vi "Main Page.vi"(8 "error in (no error)":errorcluster, 11 "Node Ptr":T1 format="%.0x") -> (0 "error out":errorcluster)   [LabVIEW 2020, in "NI PXIe-4340 System Explorer.lvlib"]
uses:
  NI PXIe-4340 System Explorer.lvlib
  <vilib>/NI VeriStand/Custom Device API/Custom Device Item Ref.ctl
  Shared/Constants.vi
  <vilib>/NI VeriStand/Custom Device API/Set Item Property (String).vi
  <vilib>/NI VeriStand/Custom Device API/Set Item Property (Double).vi
  <vilib>/NI VeriStand/Custom Device API/Set Item Property (Variant).vi
  <vilib>/NI VeriStand/Custom Device API/Custom Device API.lvlib
  Shared/NI PXIe-4340 Shared.lvlib
panel:
  in  "Sample Rate (Hz)":dbl
  in  "Device Name":string
  in  "Configure Physical Channels":bool
  in  "Header":cluster{"Section Name":string}={"Section Name"="Custom Device Item Settings"}
  in  "Description":string
  in  "Name":string
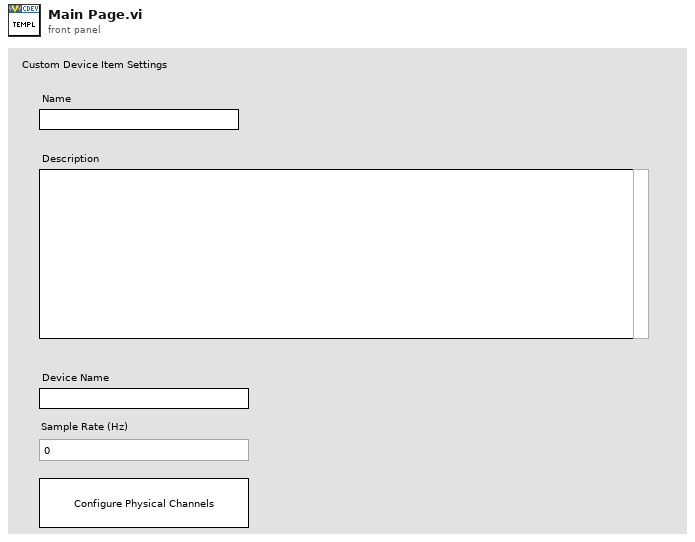
[diagram p1: front panel]
types:
  T1 = typedef "Custom Device API.lvlib/Custom Device Item Ref.ctl" = u64
  T2 = typedef "Custom Device API.lvlib/Custom Device Item Info.ctl" = cluster{"Name":string, "Is Channel":bool, "GUID":string, "Is Waveform":bool}
  T3 = typedef "NI PXIe-4340 Shared.lvlib/Device Configuration.ctl" = cluster{"Task":refnum<k21>, "Device Name":string, "Sample Rate (Hz)":dbl, "Enabled Channels":bool[]}
  T4 = typedef "Custom Device API.lvlib/Custom Device Commands.ctl" = enum16{"Default", "Item renamed", "Shutdown", "Dynamic button pressed"}
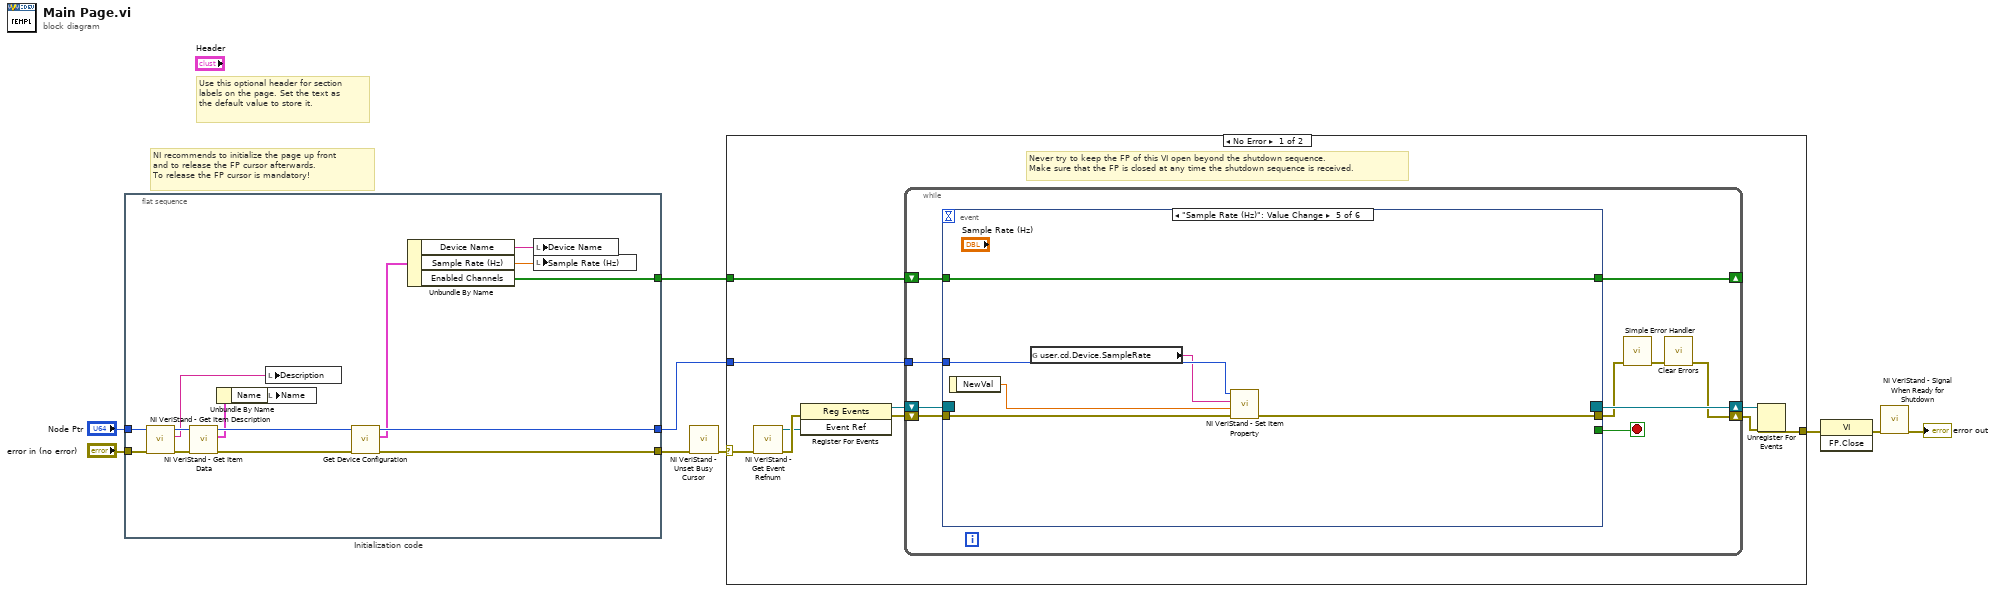
[diagram p0: block diagram]
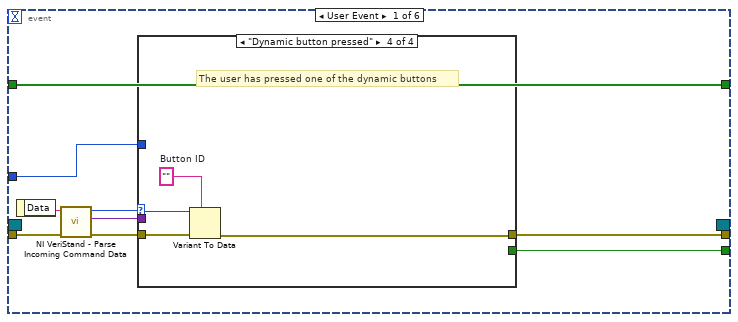
[diagram p2: hidden frame]
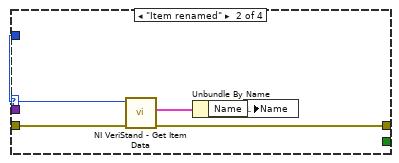
[diagram p4: hidden frame]
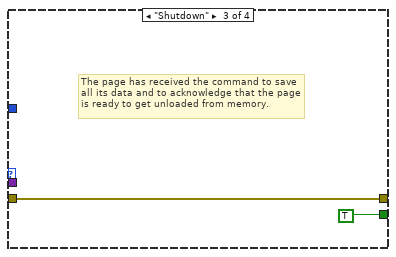
[diagram p5: hidden frame]
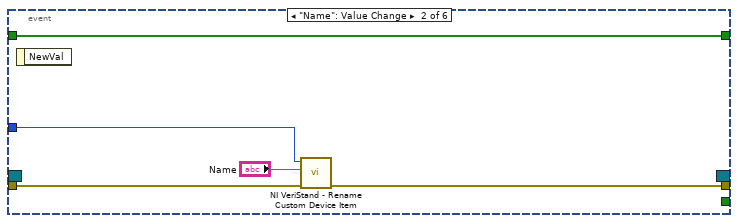
[diagram p6: hidden frame]
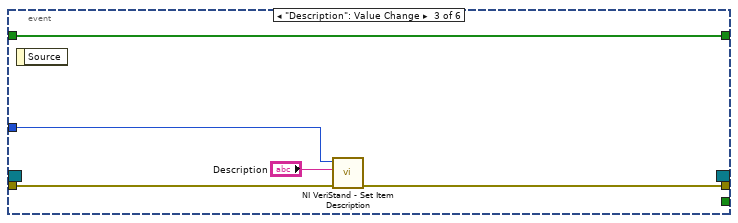
[diagram p7: hidden frame]
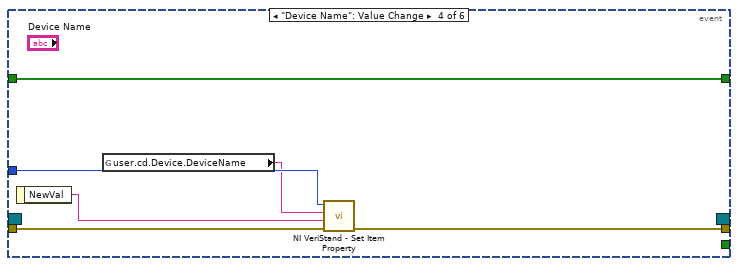
[diagram p8: hidden frame]
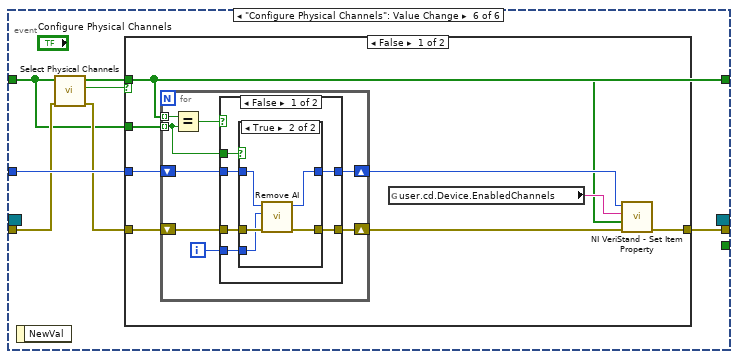
[diagram p9: hidden frame]
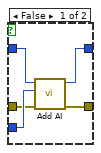
[diagram p10: hidden frame]
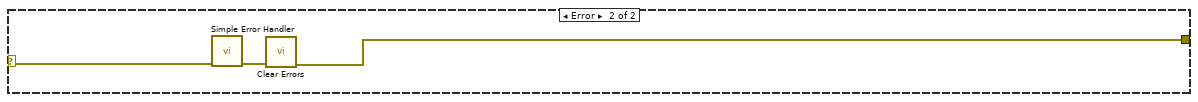
[diagram p13: hidden frame]
diagram:
  # "Use this optional header for section labels on the page. Set the text as the default value to store it."
  # "NI recommends to initialize the page up front\nand to release the FP cursor afterwards.\nTo release the FP cursor is mandatory!"
  n1 = flat-sequence "Initialization code" {
    tunnel: "error in (no error)" -> [w22]
    tunnel: "Node Ptr" -> [w21]
    tunnel: [w15] -> w5
    tunnel: [w14] -> w2
    tunnel: [w10] -> w1
    frame #0 {
      n2 = call <vilib>:"NI VeriStand - Get Item Description.vi"("error in (no error)"=w22, "Item Ref in"=w21) -> ("error out"=w19:errorcluster, "Description"=w20:string, "Item Ref out"=w23:T1)  [unwired: 7 out]
      n3 = call <vilib>:"NI VeriStand - Get Item Data.vi"("error in (no error)"=w19, "Item Ref in"=w23) -> ("error out"=w16:errorcluster, "Item Info"=w18:T2, "Item Ref out"=w24:T1)  [unwired: 7 out]
      n4 = Unbundle By Name(w18) -> ("Name"=w17:string)
      n5 = local write "Description"(w20) -> ()
      n6 = local write "Name"(w17) -> ()
      n7 = call "Get Device Configuration.vi"("error in (no error)"=w16, "Device Item Ref in"=w24) -> ("error out"=w15:errorcluster, "Device Configuration"=w13:T3, "Device Item Ref out"=w14:T1)  [unwired: 7 in]
      n8 = Unbundle By Name(w13) -> ("Device Name"=w12:string, "Sample Rate (Hz)"=w11:dbl, "Enabled Channels"=w10:bool[])
      n9 = local write "Device Name"(w12) -> ()
      n10 = local write "Sample Rate (Hz)"(w11) -> ()
    }
  }
  n11 = call <vilib>:"NI VeriStand - Unset Busy Cursor.vi"("error in (no error)"=w5) -> ("error out"=w4:errorcluster)  [unwired: 10 out]
  n12 = case shown="No Error" w4 {
    selector: w4 -> [w26 w132]
    tunnel: [w31 w130] -> w9
    tunnel: w2 -> [w27 _]
    tunnel: w1 -> [w25 _]
    frame No Error {
      # "Never try to keep the FP of this VI open beyond the shutdown sequence.\nMake sure that the FP is closed at any time the shutdown sequence is received."
      n13 = call <vilib>:"NI VeriStand - Get Event Refnum.vi"("error in (no error)"=w26) -> ("error out"=w34:errorcluster, "Event Ref"=w30:refnum<user-event>)  [unwired: 9 out]
      n14 = register-events(error in=w34, w30) -> (reference out=w28:refnum<event-registration>, error out=w29:errorcluster)  [unwired: 1 in]
      n15 = while {
        tunnel: w27 -> [w40]
        shift-right: [w37] -> w32
        shift-left: w29 -> [w43]
        shift-right: [w44] -> w33
        shift-left: w28 -> [w42]
        shift-right: [w35] -> _
        shift-left: w25 -> [w36]
        stop <- w41 stop-if-true
        n16 = event shown="[4] \"Sample Rate (Hz)\": Value Change" {
          selector: w42 -> [_ _ _ _ _ _]
          dyn-events: [_ _ _ _ _ _] -> w44
          timeout: _ -> [_ _ _ _ _ _]
          tunnel: w43 -> [w53 w70 w74 w80 w86 w91]
          tunnel: [w49 _ _ _ _ _] -> w41
          tunnel: [w48 w69 w73 w79 w85 w94] -> w39
          tunnel: w40 -> [w47 w68 w75 w78 w84 w93]
          tunnel: w36 -> [w45 w66 w71 w81 w87 w88]
          tunnel: [w45 w66 w71 w81 w87 w92] -> w35
          event User Event {
            n17 = event-data() -> ("Data"=w52:string)  [unwired: 1 out]
            n18 = call <vilib>:"NI VeriStand - Parse Incoming Command Data.vi"("error in (no error)"=w53, "Incoming data"=w52) -> ("error out"=w51:errorcluster, "Outgoing data"=w46:variant, "Action"=w50:T4)  [unwired: 7 out]
            n19 = case shown="\"Dynamic button pressed\"" w50 {
              tunnel: w51 -> [w54 w59 w60 w65]
              tunnel: [_ _ TRUE _] -> w49
              tunnel: [w54 w56 w60 w62] -> w48
              tunnel: w47 -> [_ w58 _ _]
              tunnel: w46 -> [_ _ _ w64]
              frame "Default", Default {
              }
              frame "Item renamed" {
                n20 = call <vilib>:"NI VeriStand - Get Item Data.vi"("error in (no error)"=w59, "Item Ref in"=w58) -> ("error out"=w56:errorcluster, "Item Info"=w57:T2)  [unwired: 8 out]
                n21 = Unbundle By Name(w57) -> ("Name"=w55:string)
                n22 = local write "Name"(w55) -> ()
              }
              frame "Shutdown" {
                # "The page has received the command to save all its data and to acknowledge that the page is ready to get unloaded from memory."
              }
              frame "Dynamic button pressed" {
                w63 = ""  # Button ID
                # "The user has pressed one of the dynamic buttons"
                n23 = Variant To Data(error in=w65, type=w63, Variant=w64) -> (error out=w62:errorcluster)  [unwired: 1 out]
              }
            }
          }
          event "Name": Value Change {
            n24 = event-data() -> ()  [unwired: 2 out]
            n25 = call <vilib>:"NI VeriStand - Rename Custom Device Item.vi"("error in (no error)"=w70, "New Name"="Name", "Item Ref in"=w68) -> ("error out"=w69:errorcluster)  [unwired: 1 in, 7 out]
          }
          event "Description": Value Change {
            n26 = event-data() -> ()  [unwired: 2 out]
            n27 = call <vilib>:"NI VeriStand - Set Item Description.vi"("error in (no error)"=w74, "Description"="Description", "Item Ref in"=w75) -> ("error out"=w73:errorcluster)  [unwired: 8 out]
          }
          event "Device Name": Value Change {
            n28 = event-data() -> ("NewVal"=w77:string)  [unwired: 1 out]
            n29 = global read "Constants.vi" "user.cd.Device.DeviceName"() -> (w76:string)
            n30 = call-poly <vilib>:"NI VeriStand - Set Item Property.vi"("error in (no error)"=w80, "Value"=w77, "Property Name"=w76, "Item Ref in"=w78) -> ("error out"=w79:errorcluster)  [unwired: 5 in, 2 out]
          }
          event "Sample Rate (Hz)": Value Change {
            n31 = event-data() -> ("NewVal"=w83:dbl)  [unwired: 1 out]
            n32 = global read "Constants.vi" "user.cd.Device.SampleRate"() -> (w82:string)
            n33 = call-poly <vilib>:"NI VeriStand - Set Item Property.vi"("error in (no error)"=w86, "Value"=w83, "Property Name"=w82, "Item Ref in"=w84) -> ("error out"=w85:errorcluster)  [unwired: 5 in, 2 out]
          }
          event "Configure Physical Channels": Value Change {
            n34 = event-data() -> ()  [unwired: 2 out]
            n35 = call "Select Physical Channels.vi"("error in"=w91, "Physical Channels In"=w88) -> ("error out"=w90:errorcluster, "Cancelled?"=w89:bool, "Physical Channels Out"=w92:bool[])  [unwired: 7 in]
            n36 = case shown="False" w89 {
              tunnel: [w102 w129] -> w94
              tunnel: w93 -> [w100 _]
              tunnel: w92 -> [w96 _]
              tunnel: w90 -> [w98 w129]
              tunnel: w88 -> [w95 _]
              frame False {
                n37 = for {
                  tunnel: w96 -> [w110] mode=indexing
                  tunnel: w95 -> [w106] mode=indexing
                  shift-right: [w104] -> w99
                  shift-left: w100 -> [w108]
                  shift-right: [w103] -> w97
                  shift-left: w98 -> [w107]
                  i -> [w105]
                  n38 = Equal?(x=w110, y=w106) -> (x = y?=w109:bool)
                  n39 = case shown="False" w109 {
                    tunnel: w108 -> [w114 w128]
                    tunnel: w107 -> [w113 w127]
                    tunnel: w106 -> [w116 _]
                    tunnel: w105 -> [w115 _]
                    tunnel: [w112 w128] -> w104
                    tunnel: [w111 w127] -> w103
                    frame False {
                      n40 = case shown="True" w116 {
                        tunnel: w115 -> [w120 w125]
                        tunnel: w114 -> [w121 w124]
                        tunnel: w113 -> [w119 w126]
                        tunnel: [w118 w122] -> w112
                        tunnel: [w117 w123] -> w111
                        frame False {
                          n41 = call "Add AI.vi"("error in (no error)"=w119, "Physical Channel Number"=w120, "Device Item Ref in"=w121) -> ("error out"=w117:errorcluster, "Parent Ref out"=w118:T1)  [unwired: 7 in]
                        }
                        frame True {
                          n42 = call "Remove AI.vi"("error in (no error)"=w126, "Iteration"=w125, "Item Ref in"=w124) -> ("error out"=w123:errorcluster, "Item Ref out"=w122:T1)  [unwired: 7 in]
                        }
                      }
                    }
                    frame True {
                    }
                  }
                }
                n43 = global read "Constants.vi" "user.cd.Device.EnabledChannels"() -> (w101:string)
                n44 = call-poly <vilib>:"NI VeriStand - Set Item Property.vi"("error in (no error)"=w97, "Value"=w96, "Property Name"=w101, "Item Ref in"=w99) -> ("error out"=w102:errorcluster)  [unwired: 5 in, 2 out]
              }
              frame True {
              }
            }
          }
        }
        n45 = call <vilib>:"Simple Error Handler.vi"("error in (no error)"=w39) -> ("error out"=w38:errorcluster)  [unwired: 1 in, 7 out]
        n46 = call <vilib>:"Clear Errors.vi"("error in (no error)"=w38) -> ("error out"=w37:errorcluster)  [unwired: 1 in, 5 out]
      }
      n47 = Unregister For Events(event registration refnum=w33, error in=w32) -> (error out=w31:errorcluster)
    }
    frame Error {
      n48 = call <vilib>:"Simple Error Handler.vi"("error in (no error)"=w132) -> ("error out"=w131:errorcluster)  [unwired: 1 in, 7 out]
      n49 = call <vilib>:"Clear Errors.vi"("error in (no error)"=w131) -> ("error out"=w130:errorcluster)  [unwired: 1 in, 5 out]
    }
  }
  n50 = invoke class="VI" method="FP.Close"(error in=w9) -> (error out=w8:errorcluster)  [unwired: 2 in, 2 out]
  n51 = call <vilib>:"NI VeriStand - Signal When Ready for Shutdown.vi"("error in (no error)"=w8) -> ("error out"=→"error out":errorcluster)  [unwired: 10 out]
